vi "generateModels_v2.vi"() -> ()   [LabVIEW 2016]
panel:
  in  "Scan Done?":bool
  in  "Restart":bool
  out "error IO":errorcluster
  in  "Testing only: Input SCAN_NO":string="0011"
  out "SCAN_NO":string
  out "PC Processed":bool
  out "ACh Processed":bool
  in  "Build Model":bool
  in  "Process VSCAN":bool
  in  "stop":bool
  # "You can use these pairs of vscans for testing (left column is ACh; right col is PC vscan)\nThey are paired AND ordered, meaning you must run the ACh one first, and then the corresponding PC one\nEye 1: 0032\t\t0034\nEye 2: 0035\t\t0036\nEye 3: 0037\t\t0038\nEye 4: 0040\t\t0041\nEye 5: 0043\t\t0044\nEye 6: 0046\t\t0047 << This one has a weird pupil fit; I'm still trying to figure out why\nEye 7: 0048\t\t0049"
  # ">>>"
  # ">>>"
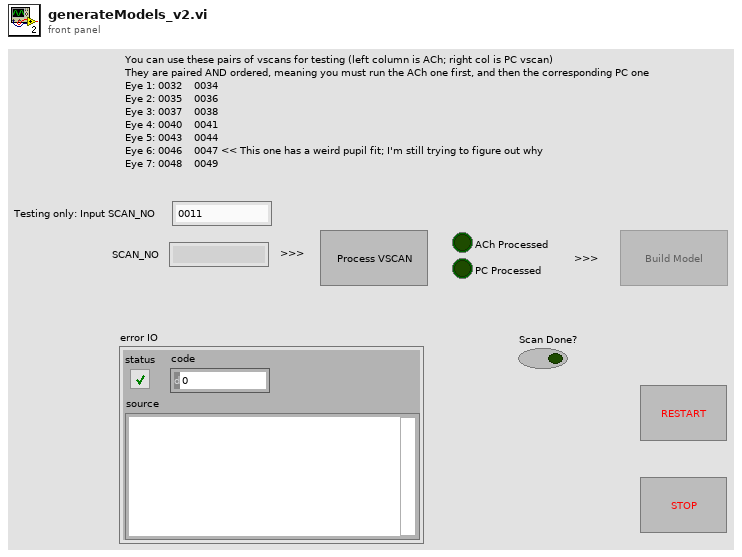
[diagram p1: front panel]
types:
  T1 = enum8{"Enabled", "Disabled", "Disabled and Grayed Out"}
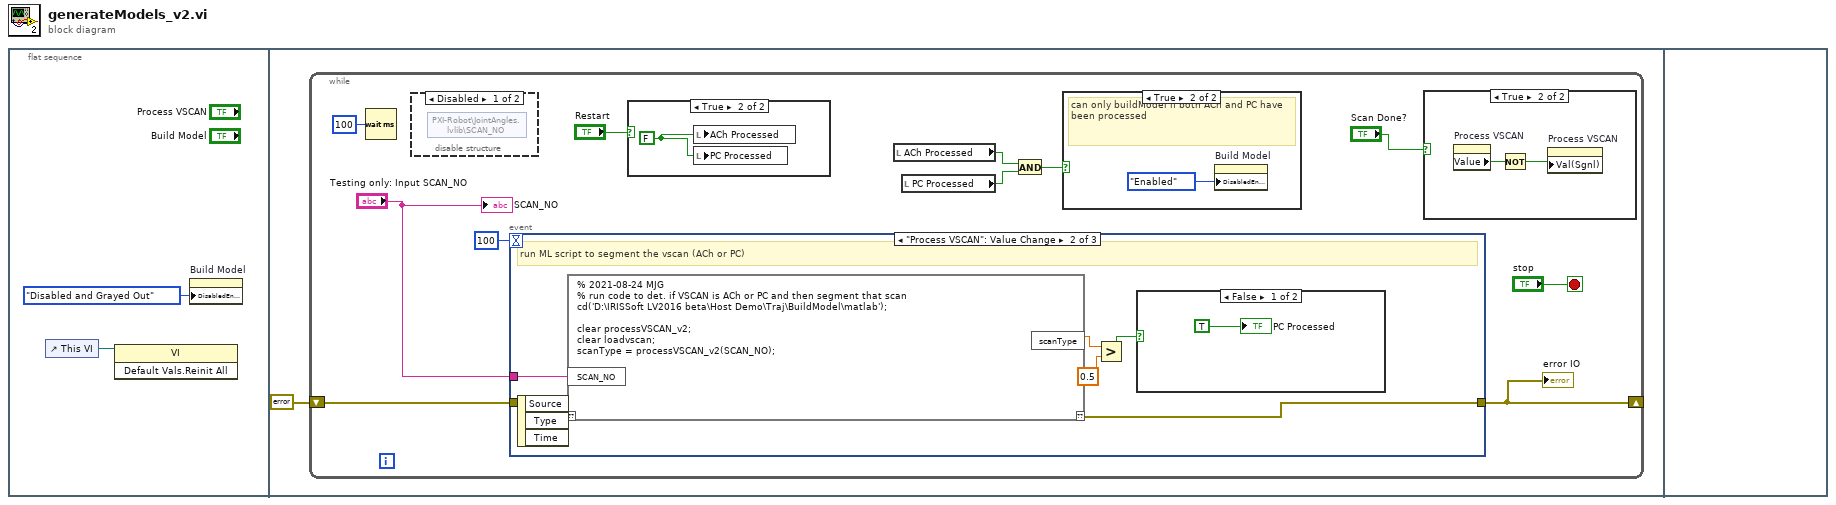
[diagram p0: block diagram]
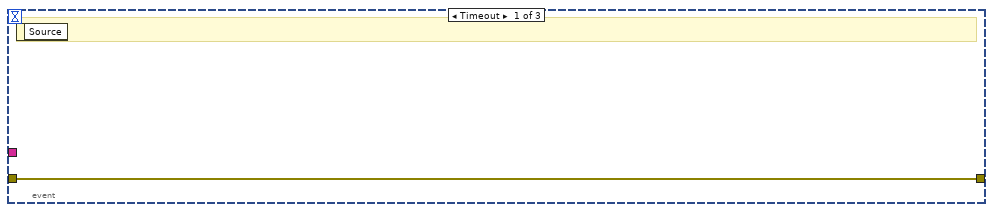
[diagram p6: hidden frame]
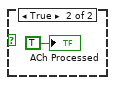
[diagram p7: hidden frame]
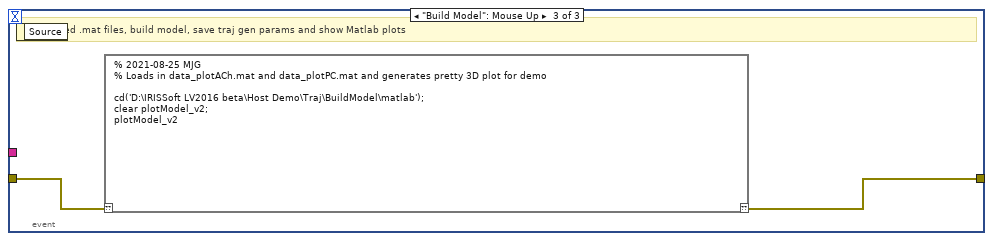
[diagram p8: hidden frame]
diagram:
  n1 = flat-sequence {
    frame #0 {
      n2 = control-ref of="This VI"() -> (w1:refnum<vi>)
      n3 = invoke class="VI" method="Default Vals.Reinit All"(reference=w1) -> ()  [unwired: 2 in, 3 out]
      n4 = property on="Build Model" class="Bool (strict)"("DisabledEnum"=T1."Disabled and Grayed Out" ("Disabled")) -> ()  [unwired: 2 in, 2 out]
    }
    frame #1 {
      n5 = while {
        shift-right: [w10] -> _
        shift-left: errorcluster {"status"=FALSE, "code"=0, "source"=""} ("error IO") -> [w9]
        stop <- "stop" stop-if-true
        n6 = Wait (ms)(milliseconds to wait=u32 100) -> ()  [unwired: 1 out]
        n7 = disable-structure shown="Disabled" {
          frame Disabled {
            n8 = shared-variable "PXI-Robot\\JointAngles.lvlib\\SCAN_NO"() -> ()  [unwired: 1 in, 2 out]
          }
          frame Enabled {
          }
        }
        n9 = event shown="[1] \"Process VSCAN\": Value Change" {
          selector: _ -> [_ _ _]
          dyn-events: _ -> [_ _ _]
          timeout: 100 -> [_ _ _]
          tunnel: "Testing only: Input SCAN_NO" -> [_ w23 _]
          tunnel: [w19 w24 w29] -> w10
          tunnel: w9 -> [w19 w25 w28]
          event Timeout {
            # "timeout"
            n10 = event-data() -> ()  [unwired: 1 in, 1 out]
          }
          event "Process VSCAN": Value Change {
            # "run ML script to segment the vscan (ACh or PC)"
            n11 = event-data() -> ()  [unwired: 1 in, 3 out]
            n12 = script code="% 2021-08-24 MJG \n% run code to det. if VSCAN is ACh or PC and then segment that scan\ncd('D:\\IRISSoft LV2016 beta\\Host Demo\\Traj\\BuildModel\\matlab');\n\nclear processVSCAN_v2;\nclear loadvscan;\nscanType = processVSCAN_v2(SCAN_NO);"("??"=w25, "SCAN_NO"=w23) -> ("??"=w24:errorcluster, "scanType"=w22:dbl)
            n13 = Greater?(x=w22, y=0.5) -> (0:w20:bool)
            n14 = case shown="False" w20 {
              frame False {
                "PC Processed" <- TRUE ("PC Processed")
              }
              frame True {
                "ACh Processed" <- TRUE ("ACh Processed")
              }
            }
          }
          event "Build Model": Mouse Up {
            # "using saved .mat files, build model, save traj gen params and show Matlab plots"
            n15 = event-data() -> ()  [unwired: 1 in, 1 out]
            n16 = script code="% 2021-08-25 MJG \n% Loads in data_plotACh.mat and data_plotPC.mat and generates pretty 3D plot for demo\n\ncd('D:\\IRISSoft LV2016 beta\\Host Demo\\Traj\\BuildModel\\matlab');\nclear plotModel_v2;\nplotModel_v2"("??"=w28) -> ("??"=w29:errorcluster)
          }
        }
        "error IO" <- w10
        n17 = case shown="True" "Restart" {
          frame False {
          }
          frame True {
            w17 = FALSE ("ACh Processed")
            n18 = local write "ACh Processed"(w17) -> ()
            n19 = local write "PC Processed"(w17) -> ()
          }
        }
        n20 = local read "ACh Processed"() -> (w13:bool)
        n21 = local read "PC Processed"() -> (w12:bool)
        n22 = And(x=w13, y=w12) -> (x .and. y?=w6:bool)
        n23 = case shown="True" w6 {
          frame False {
          }
          frame True {
            # "can only buildModel if both ACh and PC have been processed"
            n24 = property on="Build Model" class="Bool (strict)"("DisabledEnum"=T1."Enabled" ("Disabled")) -> ()  [unwired: 2 in, 2 out]
          }
        }
        n25 = case shown="True" "Scan Done?" {
          frame False {
          }
          frame True {
            n26 = property on="Process VSCAN" class="Bool (strict)"() -> ("Value"=w16:bool)  [unwired: 2 in, 2 out]
            n27 = Not(x=w16) -> (.not. x?=w15:bool)
            n28 = property on="Process VSCAN" class="Bool (strict)"("Val(Sgnl)"=w15) -> ()  [unwired: 2 in, 2 out]
          }
        }
        "SCAN_NO" <- "Testing only: Input SCAN_NO"
      }
    }
    frame #2 {
    }
  }
